vi "Post-Uninstall Custom Action.vi"(10 "Variant":variant) -> (0 "error out":errorcluster)   [LabVIEW 2020]
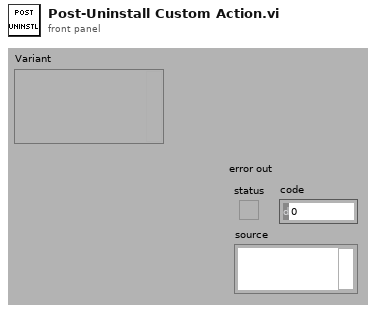
[diagram p1: front panel]
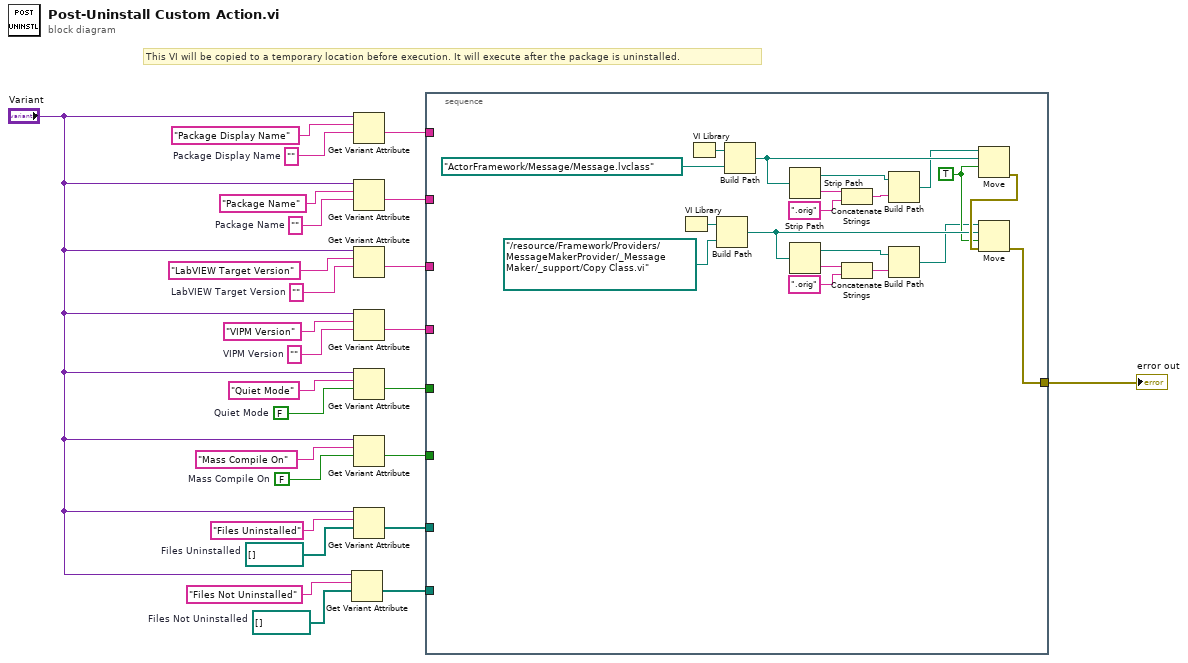
[diagram p0: block diagram]
diagram:
  w2 = path[] []  # Files Not Uninstalled
  w3 = path[] []  # Files Uninstalled
  w9 = FALSE  # Mass Compile On
  w10 = ""  # Package Display Name
  w17 = FALSE  # Quiet Mode
  w20 = ""  # VIPM Version
  w22 = ""  # LabVIEW Target Version
  w24 = ""  # Package Name
  # "This VI will be copied to a temporary location before execution. It will execute after the package is uninstalled."
  n1 = Get Variant Attribute(Variant="Variant", name="Files Not Uninstalled", default value (empty Variant)=w2) -> (value=w7:path[])  [unwired: 1 in, 3 out]
  n2 = Get Variant Attribute(Variant="Variant", name="Package Display Name", default value (empty Variant)=w10) -> (value=w16:string)  [unwired: 1 in, 3 out]
  n3 = Get Variant Attribute(Variant="Variant", name="Package Name", default value (empty Variant)=w24) -> (value=w15:string)  [unwired: 1 in, 3 out]
  n4 = Get Variant Attribute(Variant="Variant", name="LabVIEW Target Version", default value (empty Variant)=w22) -> (value=w14:string)  [unwired: 1 in, 3 out]
  n5 = Get Variant Attribute(Variant="Variant", name="VIPM Version", default value (empty Variant)=w20) -> (value=w13:string)  [unwired: 1 in, 3 out]
  n6 = Get Variant Attribute(Variant="Variant", name="Quiet Mode", default value (empty Variant)=w17) -> (value=w12:bool)  [unwired: 1 in, 3 out]
  n7 = Get Variant Attribute(Variant="Variant", name="Mass Compile On", default value (empty Variant)=w9) -> (value=w11:bool)  [unwired: 1 in, 3 out]
  n8 = Get Variant Attribute(Variant="Variant", name="Files Uninstalled", default value (empty Variant)=w3) -> (value=w6:path[])  [unwired: 1 in, 3 out]
  n9 = stacked-sequence {
    tunnel: w16 -> [_]
    tunnel: w15 -> [_]
    tunnel: w14 -> [_]
    tunnel: w13 -> [_]
    tunnel: w12 -> [_]
    tunnel: w11 -> [_]
    tunnel: w6 -> [_]
    tunnel: w7 -> [_]
    tunnel: [w27] -> w1
    frame #0 {
      w30 = TRUE ("overwrite (F)")
      n10 = VI Library() -> (path=w41:path)
      n11 = VI Library() -> (path=w44:path)
      n12 = Build Path(base path=w41, name or relative path=path "../resource/Framework/Providers/MessageMakerProvider/_Message Maker/_support/Copy Class.vi") -> (appended path=w31:path)
      n13 = Build Path(base path=w44, name or relative path=path "ActorFramework/Message/Message.lvclass") -> (appended path=w32:path)
      n14 = Strip Path(path=w32) -> (stripped path=w33:path, name=w40:string)
      n15 = Strip Path(path=w31) -> (stripped path=w34:path, name=w35:string)
      n16 = Concatenate Strings(w40, ".orig" ("string")) -> (w38:string)
      n17 = Concatenate Strings(w35, ".orig" ("string")) -> (w37:string)
      n18 = Build Path(base path=w33, name or relative path=w38) -> (appended path=w29:path)
      n19 = Build Path(base path=w34, name or relative path=w37) -> (appended path=w28:path)
      n20 = Move(source path=w29, 9:w30, 10:w32) -> (error out=w45:errorcluster)  [unwired: 2 in, 2 out]
      n21 = Move(source path=w28, error in=w45, 9:w30, 10:w31) -> (error out=w27:errorcluster)  [unwired: 1 in, 2 out]
    }
  }
  "error out" <- w1
